vi "3DF-20_Format (subVI).vi"(0 "raw (hex)":string) -> (4 "BATTERY":i32(slide) scale=0.0..3.0, 6 "X":dbl, 8 "Y":dbl, 10 "Z":dbl)   [LabVIEW 2022 SP3]
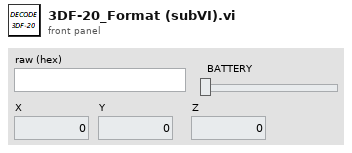
[diagram p1: front panel]
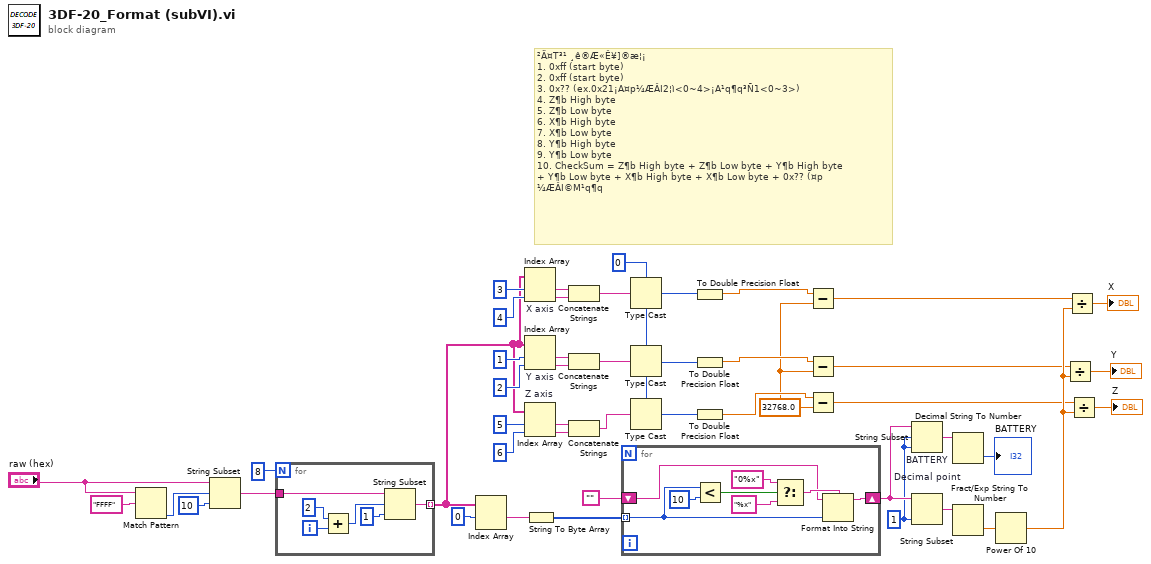
[diagram p0: block diagram]
diagram:
  w1 = 32768.0 ("y")
  w20 = 1 ("length (rest)")
  w25 = u16 0
  # "²Ä¤T³¹ ¸ê®Æ«Ê¥]®æ¦¡\n1. 0xff (start byte)\n2. 0xff (start byte)\n3. 0x?? (ex.0x21¡A¤p¼ÆÂI2¦ì<0~4>¡A¹q¶q³Ñ1<0~3>)\n4. Z¶b High byte\n5. Z¶b Low byte\n6. X¶b High byte\n7. X¶b Low byte\n8. Y¶b High byte\n9. Y¶b Low byte\n10. CheckSum = Z¶b High byte + Z¶b Low byte + Y¶b High byte \n+ Y¶b Low byte + X¶b High byte + X¶b Low byte + 0x?? (¤p\n¼ÆÂI©M¹q¶q"
  n1 = Match Pattern(string="raw (hex)", regular expression="FFFF") -> (offset past match=w45:i32)  [unwired: 1 in, 3 out]
  n2 = String Subset(string="raw (hex)", offset (0)=w45, length (rest)=10 ("length (rest)")) -> (substring=w44:string)
  n3 = for {
    N: 8 -> [_]
    tunnel: w44 -> [w53]
    tunnel: [w50] -> w35 mode=indexing
    i -> [w52]
    n4 = Add(x=2, y=w52) -> (x+y=w49:i32)
    n5 = String Subset(string=w53, offset (0)=w49, length (rest)=1 ("length (rest)")) -> (substring=w50:string)
  }
  n6 = Index Array(array=w35, index #1=0 ("index")) -> (element #1=w24:string)  [unwired: 1 in, 1 out]
  n7 = Index Array "X axis"(array=w35, index #1=3 ("index"), index #2=4 ("index")) -> (element #1=w30:string, element #2=w29:string)
  n8 = Index Array "Y axis"(array=w35, index #1=1 ("index"), index #2=2 ("index")) -> (element #1=w32:string, element #2=w31:string)
  n9 = Index Array "Z axis"(array=w35, index #1=5 ("index"), index #2=6 ("index")) -> (element #1=w33:string, element #2=w34:string)
  n10 = String To Byte Array(string=w24) -> (unsigned byte array=w23:u8[])
  n11 = Concatenate Strings(w30, w29) -> (w26:string)
  n12 = Concatenate Strings(w32, w31) -> (w27:string)
  n13 = Concatenate Strings(w33, w34) -> (w28:string)
  n14 = for {
    tunnel: w23 -> [w56] mode=indexing
    shift-right: [w54] -> w21
    shift-left: "" -> [w55]
    n15 = Less?(x=w56, y=u8 10) -> (x < y?=w60:bool)
    n16 = Select(t="0%x", s=w60, f="%x") -> (s? t:f=w57:string)
    n17 = Format Into String(format string=w57, initial string=w55, w56) -> (resulting string=w54:string)  [unwired: 1 in, 1 out]
  }
  n18 = Type Cast(type=w25, x=w26) -> (*(type *) &x=w10:u16)
  n19 = Type Cast(type=w25, x=w27) -> (*(type *) &x=w9:u16)
  n20 = Type Cast(type=w25, x=w28) -> (*(type *) &x=w8:u16)
  n21 = To Double Precision Float(number=w10) -> (double precision float=w5:dbl)
  n22 = To Double Precision Float(number=w9) -> (double precision float=w7:dbl)
  n23 = To Double Precision Float(number=w8) -> (double precision float=w6:dbl)
  n24 = Subtract(x=w5, y=w1) -> (x-y=w4:dbl)
  n25 = Subtract(x=w7, y=w1) -> (x-y=w3:dbl)
  n26 = Subtract(x=w6, y=w1) -> (x-y=w2:dbl)
  n27 = String Subset "BATTERY"(string=w21, offset (0)=w20, length (rest)=w20) -> (substring=w19:string)
  n28 = String Subset "Decimal point"(string=w21, length (rest)=w20) -> (substring=w17:string)  [unwired: 1 in]
  n29 = Decimal String To Number(string=w19) -> (number=→"BATTERY":i32)  [unwired: 2 in, 1 out]
  n30 = Fract/Exp String To Number(string=w17) -> (number=w16:dbl)  [unwired: 3 in, 1 out]
  n31 = Power Of 10(x=w16) -> (10^x=w15:dbl)
  n32 = Divide(x=w3, y=w15) -> (x/y=→"Y":dbl)
  n33 = Divide(x=w4, y=w15) -> (x/y=→"X":dbl)
  n34 = Divide(x=w2, y=w15) -> (x/y=→"Z":dbl)
